vi "globalSetUp.vi"(8 "error in":errorcluster, 11 "Single Core Acyclic Loopback in":refnum<class "Single Core Acyclic Loopback.lvclass">) -> (0 "error out":errorcluster, 3 "Single Core Acyclic Loopback out":refnum<class "Single Core Acyclic Loopback.lvclass">)   [LabVIEW 2020, in "Single Core Acyclic Loopback.lvclass"]
uses:
  Single Core Acyclic Loopback.lvclass
  niveristand-custom-device-testing-tools/VeriStandTestUtilities/VeriStandTestUtilities.lvlib
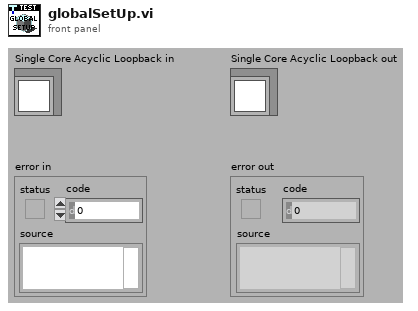
[diagram p1: front panel]
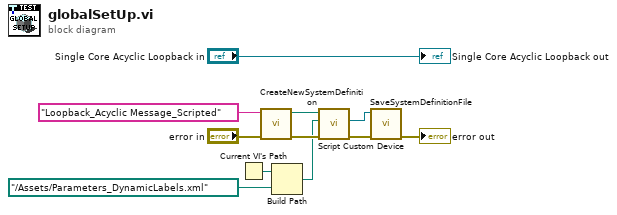
[diagram p0: block diagram]
diagram:
  n1 = Current VI's Path() -> (path=w8:path)
  n2 = call "CreateNewSystemDefinition.vi"("error in"="error in", "System Definition Name"="Loopback_Acyclic Message_Scripted" ("Channel")) -> ("error out"=w10:errorcluster, "System Definition Path"=w9:path)  [unwired: 8 in]
  n3 = Build Path(base path=w8, name or relative path=path "../Assets/Parameters_DynamicLabels.xml" ("Hardware File Path")) -> (appended path=w1:path)
  n4 = call "Script Custom Device.vi"("error in"=w10, "Parameter File Path"=w1, "System Definition File Path In"=w9) -> ("error out"=w4:errorcluster, "System Definition Reference"=w2:refnum<k24>)  [unwired: 5 in, 2 out]
  n5 = call "SaveSystemDefinitionFile.vi"("error in (no error)"=w4, "System Definition Reference in"=w2) -> ("error out"=→"error out":errorcluster)  [unwired: 8 in, 1 out]
  "Single Core Acyclic Loopback out" <- "Single Core Acyclic Loopback in"
